vi "PCO_GetDelayExposureTime.vi"(8 "error in (no error)":errorcluster, 11 "Handle":u64) -> (0 "error out":errorcluster, 1 "Exposure [s]":dbl, 2 "Delay [s]":dbl, 3 "Handle Out":u64, 5 "return type":u32 format="%x")   [LabVIEW 2011]
uses:
  SC2_Cam64.dll
panel:
  # "A00A3002 invalid Handle"
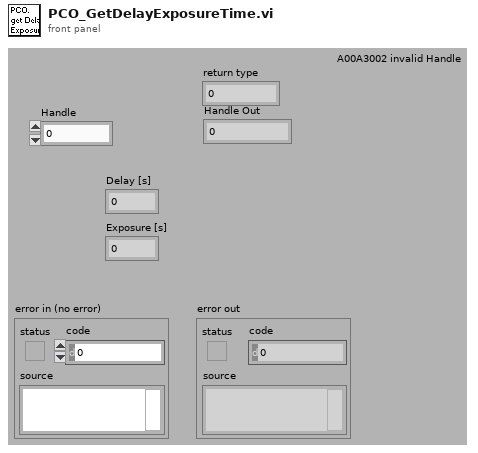
[diagram p1: front panel]
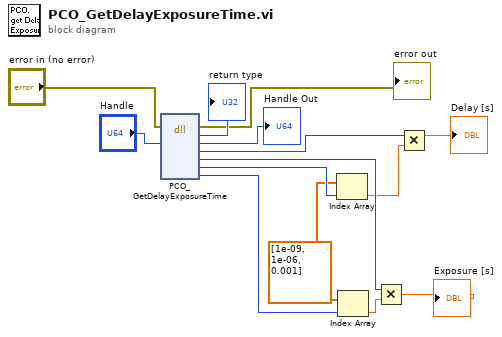
[diagram p0: block diagram]
diagram:
  w5 = dbl[] [1e-09, 1e-06, 0.001]
  n1 = dll-call lib="C:/Program Files/colibri/Drivers/PCO.Camera/SC2_Cam*.*" fn="PCO_GetDelayExposureTime"(error in="error in (no error)", "Handle"="Handle") -> (error out=→"error out":errorcluster, "return type"=→"return type":u32, "Handle"=→"Handle Out":u64, "dwDelay"=w11:u32, "dwExposure"=w8:u32, "wTimeBaseDelay"=w6:u16, "wTimeBaseExposure"=w10:u16)  [unwired: 2 in, 5 out]
  n2 = Index Array(array=w5, index=w6) -> (element=w3:dbl)
  n3 = Index Array(array=w5, index=w10) -> (element=w9:dbl)
  n4 = Multiply(x=w8, y=w9) -> (x*y=→"Exposure [s]":dbl)
  n5 = Multiply(x=w11, y=w3) -> (x*y=→"Delay [s]":dbl)
